vi "ROSRegister.vi"(0 "Err In":path, 1 "ROS to register":T3={"topic port"=0, "Node"="", "topic"="", "type"="", "node port"=0, "error "={"status"=FALSE, "code"=0, "source"=""}, "Direction"=enum."Node", "APIs"=[], "Update (ms)"=1, "write queue"=1}) -> (2 "Err Out":path, 3 "Response":T2, 4 "MyState":T5, 5 "Log":T1)   [LabVIEW 2012]
uses:
  <userlib>/ROSforLV/ROS/Code/Console/Servers/ServerSubs/MyState.ctl
  <userlib>/ROSforLV/ROS/Code/SubVIs/_ROSControl.ctl
  <userlib>/ROSforLV/ROS/Code/SubVIs/_ROSDirection.ctl
  <userlib>/ROSforLV/ROS/Code/Console/Servers/ServerSubs/ROSLog.ctl
  <userlib>/ROSforLV/ROS/Code/_ROSDefinition.vi
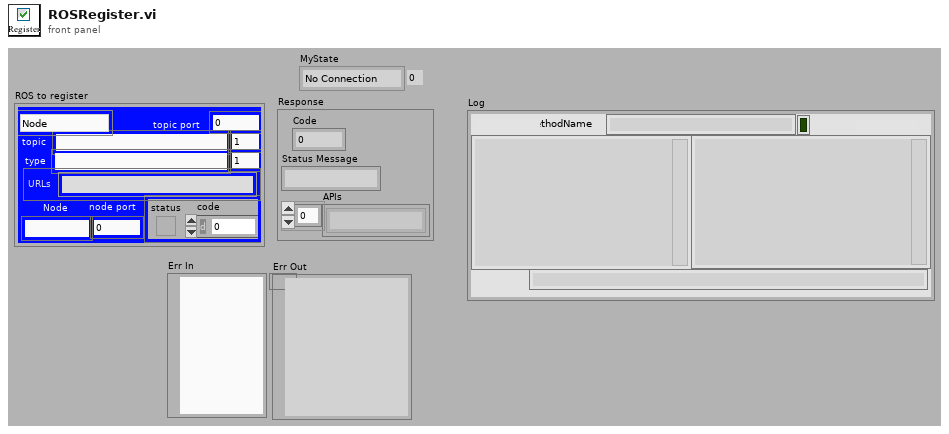
[diagram p1: front panel]
types:
  T1 = typedef "ROSLog.ctl" = cluster{"Sent":string, "Reply":string, "MethodName":string, "success":bool, "Dir1":string, "Dir2":string, "Time Stamp":string, "error":errorcluster, "Preamble":string}
  T2 = cluster{"Code":i32, "Status Message":string, "APIs":string[]}
  T3 = typedef "_ROSControl.ctl" = cluster{"topic port":u16, "Node":string, "topic":string, "type":string, "node port":u32, "error ":errorcluster, "Direction":T4, "APIs":string[], "Update (ms)":u16, "write queue":u16}
  T4 = typedef "_ROSDirection.ctl" = enum16{"Node", "Publisher", "Subscriber", "Service Client"}
  T5 = typedef "MyState.ctl" = enum16{"No Connection", "Registered", "Connected", "Close"}
  T6 = enum16{"Reset Log", "Add Client", "Remove Client", "Add Task"}
  T7 = enum16{"http://IP:port", "http://IP", "IP:port", "IP only"}
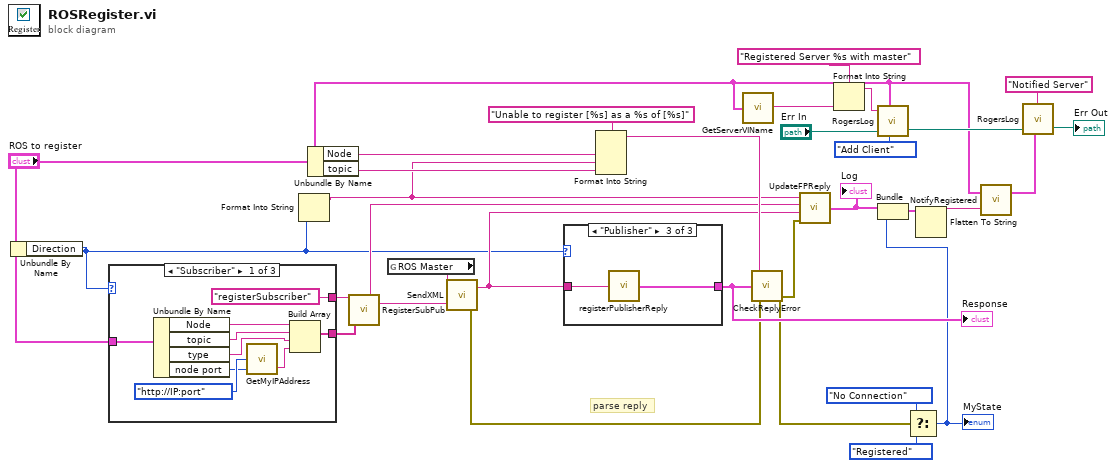
[diagram p0: block diagram]
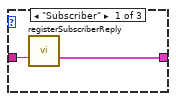
[diagram p2: hidden frame]
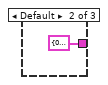
[diagram p3: hidden frame]
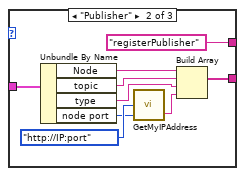
[diagram p4: hidden frame]
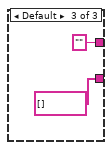
[diagram p5: hidden frame]
diagram:
  # "parse reply"
  n1 = Unbundle By Name("ROS to register") -> ("Direction"=w16:T4)
  n2 = case shown="\"Subscriber\"" w16 {
    tunnel: "ROS to register" -> [w34 w40 _]
    tunnel: ["registerSubscriber" ("MethodName") "registerPublisher" ("MethodName") "" ("MethodName")] -> w18
    tunnel: [w33 w41 string[] []] -> w17
    frame "Subscriber" {
      n3 = Unbundle By Name(w34) -> ("Node"=w38:string, "topic"=w37:string, "type"=w36:string, "node port"=w31:u32)
      n4 = call <userlib>:"GetMyIPAddress.vi"("Port"=w31, "Format"=T7."http://IP:port") -> ("URI"=w35:string)  [unwired: 2 in]
      n5 = Build Array(w38, w37, w36, w35) -> (w33:string[])
    }
    frame "Publisher" {
      n6 = Unbundle By Name(w40) -> ("Node"=w47:string, "topic"=w46:string, "type"=w45:string, "node port"=w44:u32)
      n7 = call <userlib>:"GetMyIPAddress.vi"("Port"=w44, "Format"=T7."http://IP:port") -> ("URI"=w43:string)  [unwired: 2 in]
      n8 = Build Array(w47, w46, w45, w43) -> (w41:string[])
    }
    frame Default {
    }
  }
  n9 = Format Into String(w16) -> (resulting string=w20:string)  [unwired: 3 in, 1 out]
  n10 = Unbundle By Name("ROS to register") -> ("Node"=w23:string, "topic"=w28:string)
  n11 = call <userlib>:"RegisterSubPub.vi"("Parameters"=w17, "MethodName"=w18) -> ("XML"=w19:string)
  n12 = global read "_ROSDefinition.vi" "ROS Master"() -> (w29:string)
  n13 = call <userlib>:"SendXML.vi"("Send"=w19, "URI in"=w29) -> ("error out"=w25:errorcluster, "Reply"=w21:string)
  n14 = case shown="\"Publisher\"" w16 {
    tunnel: [w51 T2 {"Code"=0, "Status Message"="", "APIs"=[]} ("Response") w55] -> w30
    tunnel: w21 -> [w52 _ w54]
    frame "Subscriber" {
      n15 = call <userlib>:"registerSubscriberReply.vi"("Response"=w52) -> ("Response"=w51:T2)
    }
    frame Default {
    }
    frame "Publisher" {
      n16 = call <userlib>:"registerPublisherReply.vi"("Response"=w54) -> ("Response"=w55:T2)
    }
  }
  "Response" <- w30
  n17 = Format Into String(format string="Unable to register [%s] as a %s of [%s]", w23, w20, w28) -> (resulting string=w24:string)  [unwired: 2 in, 1 out]
  n18 = call <userlib>:"GetServerVIName.vi"("ROS"="ROS to register") -> ("vi name"=w2:string)
  n19 = call <userlib>:"CheckReplyError.vi"("error in"=w25, "Response"=w30, "Error String"=w24) -> ("error out"=w11:errorcluster)  [unwired: 2 out]
  n20 = call <userlib>:"UpdateFPReply.vi"("error in (no error)"=w11, "Reply"=w21, "Sent"=w19, "method"=w20) -> ("Log"=w14:T1)
  "Log" <- w14
  n21 = Format Into String(format string="Registered Server %s with master" ("Text to add"), w2) -> (resulting string=w4:string)  [unwired: 2 in, 1 out]
  n22 = call <userlib>:"RogersLog.vi"("Text to add"=w4, "ROS"="ROS to register", "LogPath in"="Err In", "Task"=T6."Add Client") -> ("LogPath out"=w8:path)  [unwired: 1 in, 1 out]
  n23 = Select(t=MyState."No Connection" ("MyState"), s=w11, f=MyState."Registered" ("MyState")) -> (s? t:f=w13:T5)
  "MyState" <- w13
  n24 = Bundle("Log"=w14, "MyState"=w13) -> (w15:cluster{"Log":T1, "MyState":T5})  [unwired: 1 in]
  n25 = Flatten To String(anything=w15) -> (data string=w12:string)  [unwired: 3 in, 2 out]
  n26 = call <userlib>:"NotifyRegistered.vi"("data string"=w12, "ROS"="ROS to register") -> ("ROS out"=w6:T3)  [unwired: 1 in]
  n27 = call <userlib>:"RogersLog.vi"("Text to add"="Notified Server", "ROS"=w6, "LogPath in"=w8) -> ("LogPath out"=→"Err Out":path)  [unwired: 2 in, 1 out]
